vi "Verificar login.vi"(4 "error in (no error)":errorcluster, 5 "Password":string, 6 "Login":string, 7 "Table":string[][](array[string])=[["admin", "labview"], ["user 1", "12345"], ["guest", ""]]) -> (0 "error out":errorcluster, 3 "Verificado":bool)   [LabVIEW 2021]
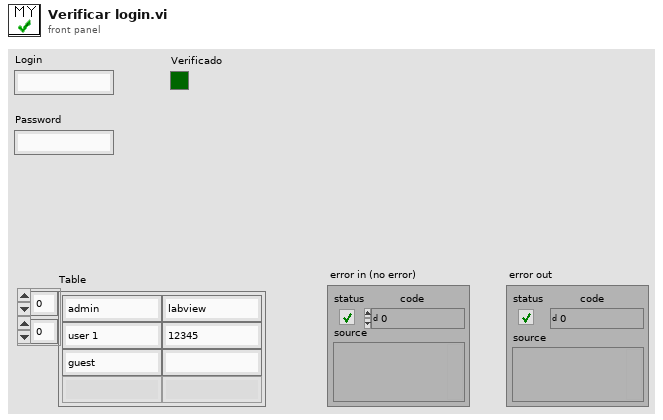
[diagram p1: front panel]
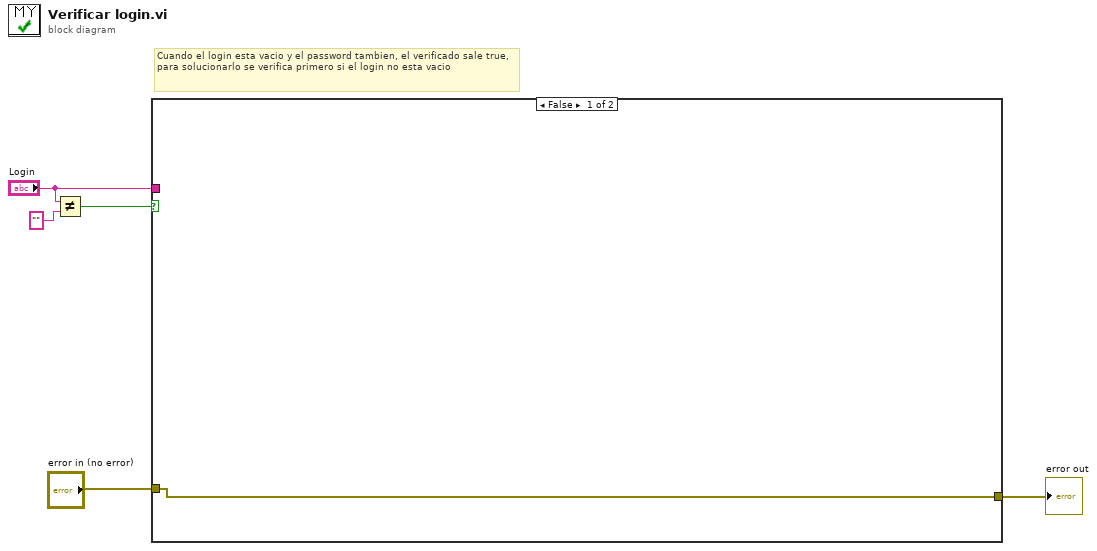
[diagram p0: block diagram]
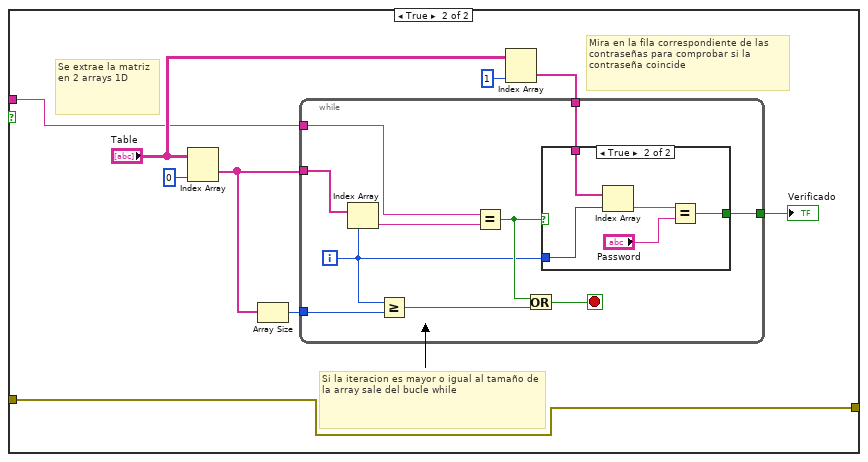
[diagram p2: hidden frame]
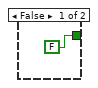
[diagram p3: hidden frame]
diagram:
  # "Cuando el login esta vacio y el password tambien, el verificado sale true, para solucionarlo se verifica primero si el login no esta vacio"
  n1 = Not Equal?(x="Login", y="") -> (x != y?=w4:bool)
  n2 = case shown="False" w4 {
    tunnel: "Login" -> [_ w8]
    tunnel: [w6 w7] -> w2
    tunnel: "error in (no error)" -> [w6 w7]
    frame False {
    }
    frame True {
      # "Mira en la fila correspondiente de las contraseñas para comprobar si la contraseña coincide"
      # "Si la iteracion es mayor o igual al tamaño de la array sale del bucle while"
      # "Se extrae la matriz en 2 arrays 1D"
      n3 = Index Array(array="Table", index (col)=0) -> (element=w11:string[])  [unwired: 1 in]
      n4 = Array Size(array=w11) -> (size(s)=w10:i32)
      n5 = Index Array(array="Table", index (col)=1) -> (element=w9:string[])  [unwired: 1 in]
      n6 = while {
        tunnel: w11 -> [w25]
        tunnel: w10 -> [w23]
        tunnel: w9 -> [w19]
        tunnel: [w18] -> w15
        tunnel: w8 -> [w16]
        i -> [w20]
        stop <- w17 stop-if-true
        n7 = Index Array(array=w25, index=w20) -> (element=w24:string)
        n8 = Greater Or Equal?(x=w20, y=w23) -> (x >= y?=w22:bool)
        n9 = Equal?(x=w16, y=w24) -> (x = y?=w21:bool)
        n10 = Or(x=w21, y=w22) -> (x .or. y?=w17:bool)
        n11 = case shown="True" w21 {
          tunnel: w20 -> [_ w31]
          tunnel: w19 -> [_ w30]
          tunnel: [FALSE w27] -> w18
          frame False {
          }
          frame True {
            n12 = Index Array(array=w30, index=w31) -> (element=w29:string)
            n13 = Equal?(x=w29, y="Password") -> (x = y?=w27:bool)
          }
        }
      }
      "Verificado" <- w15
    }
  }
  "error out" <- w2
